vi "Get.vi"(8 "error in (no error)":errorcluster, 11 "CellClick in":refnum<class "CellClick.lvclass">) -> (0 "error out":errorcluster, 3 "CellClick out":refnum<class "CellClick.lvclass">)   [LabVIEW 2014, in "DataGrid.lvlib" / "CellClick.lvclass"]
uses:
  CellClick.lvclass
  Abstract EVENT/Abstract EVENT.lvclass
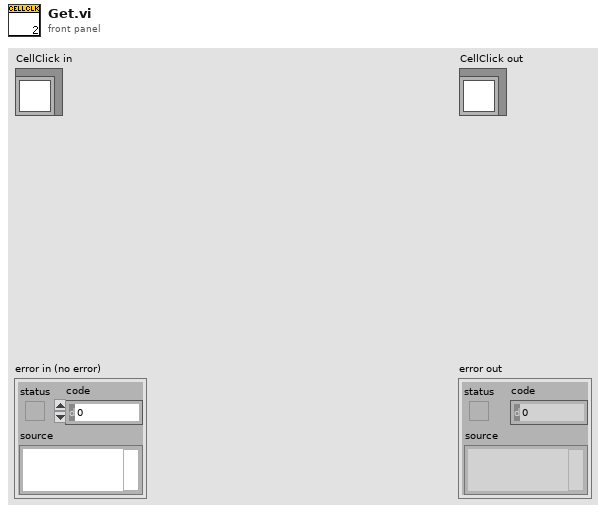
[diagram p1: front panel]
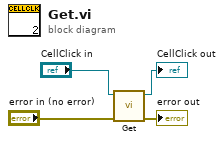
[diagram p0: block diagram]
diagram:
  n1 = call-parent "Get.vi"("error in (no error)"="error in (no error)", "Abstract EVENT in"="CellClick in") -> ("error out"=→"error out":errorcluster, "Abstract EVENT out"=→"CellClick out":refnum<class "CellClick.lvclass">)  [unwired: 8 in]
